vi "GetParametrPoly.vi"   [LabVIEW 2010, in "StepMotor.lvclass"]
uses:
  StepMotor.lvclass
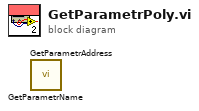
[diagram p0: block diagram]
diagram:
  n1 = call "GetParametrName.vi"() -> ()  [unwired: 9 in, 3 out]
  n2 = call "GetParametrAddress.vi"() -> ()  [unwired: 9 in, 3 out]
